vi "BSONObjectProbe.vi"(11 "response":refnum<class "tBSONDocument.lvclass">) -> (2 "JSON String":string, 3 "Boolean":bool)   [LabVIEW 2013, in "BSON.lvlib" / "tBSONDocument.lvclass"]
uses:
  tBSONDocument/tBSONDocument.lvclass
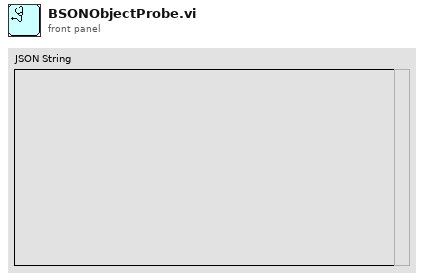
[diagram p1: front panel]
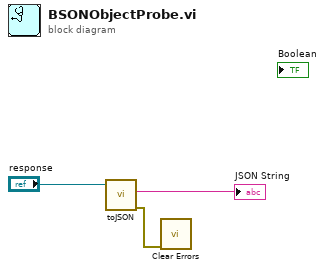
[diagram p0: block diagram]
diagram:
  n1 = call-dynamic "toJSON.vi"("tBSONDocument in"="response") -> ("error out"=w3:errorcluster, "JSON"=→"JSON String":string)  [unwired: 8 in, 1 out]
  n2 = call <vilib>:"Clear Errors.vi"("error in (no error)"=w3) -> ()  [unwired: 6 in, 1 out]
